vi "Galvo Module_sync.vi"(5 "sample mode":i32(ring)=10178 items=["Finite Samples"=10178, "Continuous Samples"=10123, "Hardware Timed Single Point"=12522], 7 "Action":T23=enum."Init: Calc scan pattern", 8 "error in (no error)":errorcluster, 10 "System Parameters":T1={"Optical Parameters"={"Obj. Focal Length [mm]"=45.0, "Scan Lens EFL[mm]"=60.0, "Tube Lens EFL[mm]"=180.0, "Galvo V Range (+/-)"=10.0, "Galvo Max Half Angle [Deg]"=19.0, "Max Galvo Range[%]"=0.0}, "Vibratome"={"Pre Cut Dwell [s]"=0.0, "Blade Frequency [RPM]"=0, "Slice Speed [mm/s]"=0.0, "Post Cut Dwell [s]"=0.0, "Ramp Time [s]"=0.0, "Start X [mm]"=0.0, "Start Y [mm]"=0.0, "Slice Length [mm]"=0.0, "Slice Axis"=enum."Y Axis", "Controller VISA Ref"="COM4"}, "Table Stages"={"X Stage"={"Position"=0.0, "Is.Enabled?"=FALSE, "Is.Connected?"=FALSE, "Device SN"="45876539", "AccelerationMaximum"=0.0, "VelocityMaximum"=0.0, "Acceleration"=0.0, "Velocity"=0.0, "waitTimeout (ms)"=0, "Model"=enum."None", "Is.Homed?"=FALSE, "MOVE"=FALSE}, "Y Stage"={"Position"=0.0, "Is.Enabled?"=FALSE, "Is.Connected?"=FALSE, "Device SN"="45876539", "AccelerationMaximum"=0.0, "VelocityMaximum"=0.0, "Acceleration"=0.0, "Velocity"=0.0, "waitTimeout (ms)"=0, "Model"=enum."None", "Is.Homed?"=FALSE, "MOVE"=FALSE}, "Z Stage"={"Position"=0.0, "Is.Enabled?"=FALSE, "Is.Connected?"=FALSE, "Device SN"="45876539", "AccelerationMaximum"=0.0, "VelocityMaximum"=0.0, "Acceleration"=0.0, "Velocity"=0.0, "waitTimeout (ms)"=0, "Model"=enum."None", "Is.Homed?"=FALSE, "MOVE"=FALSE}, "Attenuator"={"Position"=0.0, "Is.Enabled?"=FALSE, "Is.Connected?"=FALSE, "Device SN"="45876539", "AccelerationMaximum"=0.0, "VelocityMaximum"=0.0, "Acceleration"=0.0, "Velocity"=0.0, "waitTimeout (ms)"=0, "Model"=enum."None", "Is.Homed?"=FALSE, "MOVE"=FALSE}}, "Imaging Parameter"={"Raster Scan Direction"=enum."Uni Directional", "Pixel Dwell Time [Clock Cycles]"=1, "Flyback Time [Clock Cycles]"=10, "XY Center [um]"={"X"=1.0, "Y"=1.0}, "Pixel Step Size [um] X"=50.0, "XY Image Size"=enum."256 x 256", "Custom"=TRUE, "Custom Size"={"X"=10, "Y"=10}, "Line Averages"=1, "Pixel Step Size [um] Y"=0.0}, "Galvo HW Parameters"={"Analog Out Channel"="GalvoCtrl/ao0,GalvoCtrl/ao1", "Min Voltage"=-10.0, "Max Voltage"=10.0, "Pixel Clock Source"="/GalvoCtrl/PFI0", "Sample Rate"=1000.0, "Line Clock Out Ch"="GalvoCtrl/port0/line0", "2P ready check"="GalvoCtrl/port0/line0"}, "Alazar parameters"={"Trigger Settings"={"General Trigger Settings"={"Trigger Operation"=0, "Coupling ID"=2, "Range ID"=2, "Delay"=0, "Timeout Ticks"=0, "Mode"=1, "Parameter"=1}, "Trigger Engine 1"={"Trigger Engine"=0, "Source"=2, "Slope"=1, "Level"=140}, "Trigger Engine 2"={"Trigger Engine"=1000, "Source"=4294967295, "Slope"=1, "Level"=2048}}, "Device ID"={"System ID"=1, "Board ID"=1}, "Ch A Input Control"={"Channel"=1, "Coupling"=2, "Range"=10, "Impedance"=2}, "Ch B Input Control"={"Channel"=2, "Coupling"=2, "Range"=10, "Impedance"=2}, "Acq Settings"={"Record Length"=1440, "Offset"=0, "Records Per Buffer"=2048, "Records Count (Records/Acq)"=2147483647, "Window Type"=1, "Footer"=0, "Samples per record"=2048, "Output Format"=257}, "Capture Clock"={"Sample Rate"=100, "Decimation"=0, "Source"=2, "Edge"=0}}, "Mosaic Paramter"={"X Axis"={"Start [mm]"=0.0, "Steps [pts]"=0.0, "End [mm]"=0.0}, "Y Axis"={"Start [mm]"=0.0, "Steps [pts]"=0.0, "End [mm]"=0.0}, "Scan Pattern"=enum."Uni-directional", "Overlap Options"={"Overlap Type"=enum."No Overlap", "Percent Overlap"=0, "Justify"=enum."Start"}}, "Manual Controls"={"Data Path"=path "", "Save parameters"={"start pixel"=45, "#pixels to save"=100}, "Acquisition mode"=enum."Alazar FFT", "PSOCT Channel"=1, "Save data?"=FALSE, "AIP rotation angle"=0.0, "Outgoing Mail Server (SMTP)"="smtp.gmail.com", "Email"="", "Password"="", "Carrier 1"=enum."Sprint", "phone number 1"="", "Subject"="", "Message"="", "Carrier 2"=enum."Sprint", "phone number 2"="", "Outputs for GPU FFT"=enum."Amp + Phase diff", "First Slice #"=1}, "Z stage setting"={"first cut height(mm)"=45.85, "cut thickness[um]"=[], "#cycles"=111, "PSOCT thickness(um)"=[], "First image height(mm)"=2.1, "Pause?"=[], "Z0"=0.0, "fixed Z0?"=FALSE, "Cut_aft_2P?(leave empty if no 2P)"=[], "2P thickness(um) (leave empty if not used)"=[], "2P_cover_all_depth? (leave empty if no 2P)"=[]}, "Attenuator"={"Power after Objective (recalibrate every 6 month)"=[]}, "Pause?"=FALSE} {"Manual Controls"."PSOCT Channel" items=["A"=1, "B"=2, "A + B"=3, "C"=4, "A + C"=5, "A + B"=6, "D"=8, "A + D"=9, "B + D"=10, "C + D"=12, "A + B + C + D"=15]; "Alazar parameters"."Capture Clock"."Edge" items=["Rising", "Falling"]; "Alazar parameters"."Capture Clock"."Source" items=["Internal"=1, "Fast External"=2, "Medium External"=3, "Slow External"=4, "External AC"=5, "External DC"=6, "External 10MHz"=7]; "Alazar parameters"."Acq Settings"."Output Format" items=["Float Log"=11, "Float Amp"=10, "U16_LOG"=1, "U16_AMP2"=257, "Real"=3, "Imag"=4]; "Alazar parameters"."Acq Settings"."Footer" items=["FOOTER_NONE", "FOOTER_NPT"]; "Alazar parameters"."Acq Settings"."Window Type" items=["DSP_WINDOW_NONE", "DSP_WINDOW_HANNING", "DSP_WINDOW_HAMMING", "DSP_WINDOW_BLACKMAN", "DSP_WINDOW_BLACKMAN_HARRIS", "DSP_WINDOW_BARTLETT"]; "Alazar parameters"."Ch B Input Control"."Channel" items=["A"=1, "B"=2, "C"=4, "D"=8]; "Alazar parameters"."Ch B Input Control"."Coupling" items=["AC"=1, "DC"=2]; "Alazar parameters"."Ch B Input Control"."Range" items=["20 mV"=1, "40 mV"=2, "50 mV"=3, "80 mV"=4, "100 mV"=5, "200 mV"=6, "400 mV"=7, "500 mV"=8, "800 mV"=9, "1 V"=10, "1.25 V"=33, "2 V"=11, "4 V"=12, "5 V"=13, "8 V"=14, "10 V"=15, "20 V"=16]; "Alazar parameters"."Ch B Input Control"."Impedance" items=["1 MOhm"=1, "50 Ohm"=2, ""=0]; "Alazar parameters"."Ch A Input Control"."Channel" items=["A"=1, "B"=2, "C"=4, "D"=8]; "Alazar parameters"."Ch A Input Control"."Coupling" items=["AC"=1, "DC"=2]; "Alazar parameters"."Ch A Input Control"."Range" items=["20 mV"=1, "40 mV"=2, "50 mV"=3, "80 mV"=4, "100 mV"=5, "200 mV"=6, "400 mV"=7, "500 mV"=8, "800 mV"=9, "1 V"=10, "1.25 V"=33, "2 V"=11, "4 V"=12, "5 V"=13, "8 V"=14, "10 V"=15, "20 V"=16]; "Alazar parameters"."Ch A Input Control"."Impedance" items=["1 MOhm"=1, "50 Ohm"=2, ""=0]; "Alazar parameters"."Trigger Settings"."General Trigger Settings"."Trigger Operation" items=["J", "K", "J OR K", "J AND K", "J XOR K", "J AND NOT K", "NOT J AND K"]; "Alazar parameters"."Trigger Settings"."General Trigger Settings"."Coupling ID" items=["AC"=1, "DC"=2]; "Alazar parameters"."Trigger Settings"."General Trigger Settings"."Range ID" items=["5 V", "1 V", "TTL"]; "Alazar parameters"."Trigger Settings"."Trigger Engine 1"."Trigger Engine" items=["J", "K"]; "Alazar parameters"."Trigger Settings"."Trigger Engine 1"."Source" items=["A", "B", "External", "Disable", "C", "D"]; "Alazar parameters"."Trigger Settings"."Trigger Engine 1"."Slope" items=["Positive"=1, "Negative"=2]; "Alazar parameters"."Trigger Settings"."Trigger Engine 2"."Trigger Engine" items=["J", "K"]; "Alazar parameters"."Trigger Settings"."Trigger Engine 2"."Source" items=["A", "B", "External", "Disable", "C", "D"]; "Alazar parameters"."Trigger Settings"."Trigger Engine 2"."Slope" items=["Positive"=1, "Negative"=2]; "Imaging Parameter"."Pixel Step Size [um] Y" min=0.0 max=100.0 step=0.01; "Imaging Parameter"."Line Averages" min=1 max=30 step=1; "Imaging Parameter"."Flyback Time [Clock Cycles]" max=10 step=1; "Imaging Parameter"."Pixel Step Size [um] X" min=0.0 max=100.0 step=0.01; "Imaging Parameter"."Custom Size"."Y" min=1 max=30 step=1; "Imaging Parameter"."Custom Size"."X" min=1 max=30 step=1; "Imaging Parameter"."XY Center [um]"."Y" min=1.0 max=30.0 step=1.0; "Imaging Parameter"."XY Center [um]"."X" min=1.0 max=30.0 step=1.0; "Imaging Parameter"."Pixel Dwell Time [Clock Cycles]" max=10 step=1}) -> (0 "error out":errorcluster, 1 "task done?":bool)   [LabVIEW 2018]
uses:
  type defines/Galvo controls.ctl
  Controls/System Parameters.ctl
  Controls/Optical Parameters.ctl
  Controls/Vibratome Parameters.ctl
  Controls/Translation Stage Parameters.ctl
  Hardware Mfg/Thorlabs Translation Stages/Controls/Translation Stage Cluster.ctl
  Controls/Translation Stage Types.ctl
  Controls/Imaging Parameters.ctl
  Controls/Scan Direction.ctl
  type defines/Alazar parameters.ctl
  Hardware Mfg/AlazarTech SDK/Controls/General Trigger Settings.ctl
  Hardware Mfg/AlazarTech SDK/Controls/Trigger Engine Controls.ctl
  Hardware Mfg/AlazarTech SDK/Controls/Alazar Device ID.ctl
  Hardware Mfg/AlazarTech SDK/Controls/Channel Input Controls.ctl
  Hardware Mfg/AlazarTech SDK/Controls/Alazar Acquisition Settings.ctl
  Hardware Mfg/AlazarTech SDK/Controls/Clock Controls.ctl
  type defines/Mosaic Parameter.ctl
  type defines/Manual Controls.ctl
  type defines/FFT parameters.ctl
  type defines/FFT mode.ctl
  type defines/GPU FFT outputs.ctl
  type defines/Vibratome Param.ctl
  type defines/attenuator.ctl
  <vilib>/DAQmx/write.llb/DAQmx Write (Digital 1D U32 1Chan NSamp).vi
  <vilib>/DAQmx/write.llb/DAQmx Write (Analog 2D DBL NChan NSamp).vi
  <vilib>/DAQmx/create/channels.llb/DAQmx Create Channel (CO-Pulse Generation-Time).vi
  <vilib>/DAQmx/create/channels.llb/DAQmx Create Channel (AO-Voltage-Basic).vi
  <vilib>/DAQmx/configure/timing.llb/DAQmx Timing (Sample Clock).vi
  <vilib>/DAQmx/create/channels.llb/DAQmx Create Channel (DO-Digital Output).vi
  <vilib>/DAQmx/configure/trigger.llb/DAQmx Start Trigger (Digital Edge).vi
  <vilib>/DAQmx/miscellaneous.llb/DAQmx Fill In Error Info.vi
  <resource>/objmgr/daqmx.rc
panel:
  # "X"
  # "X"
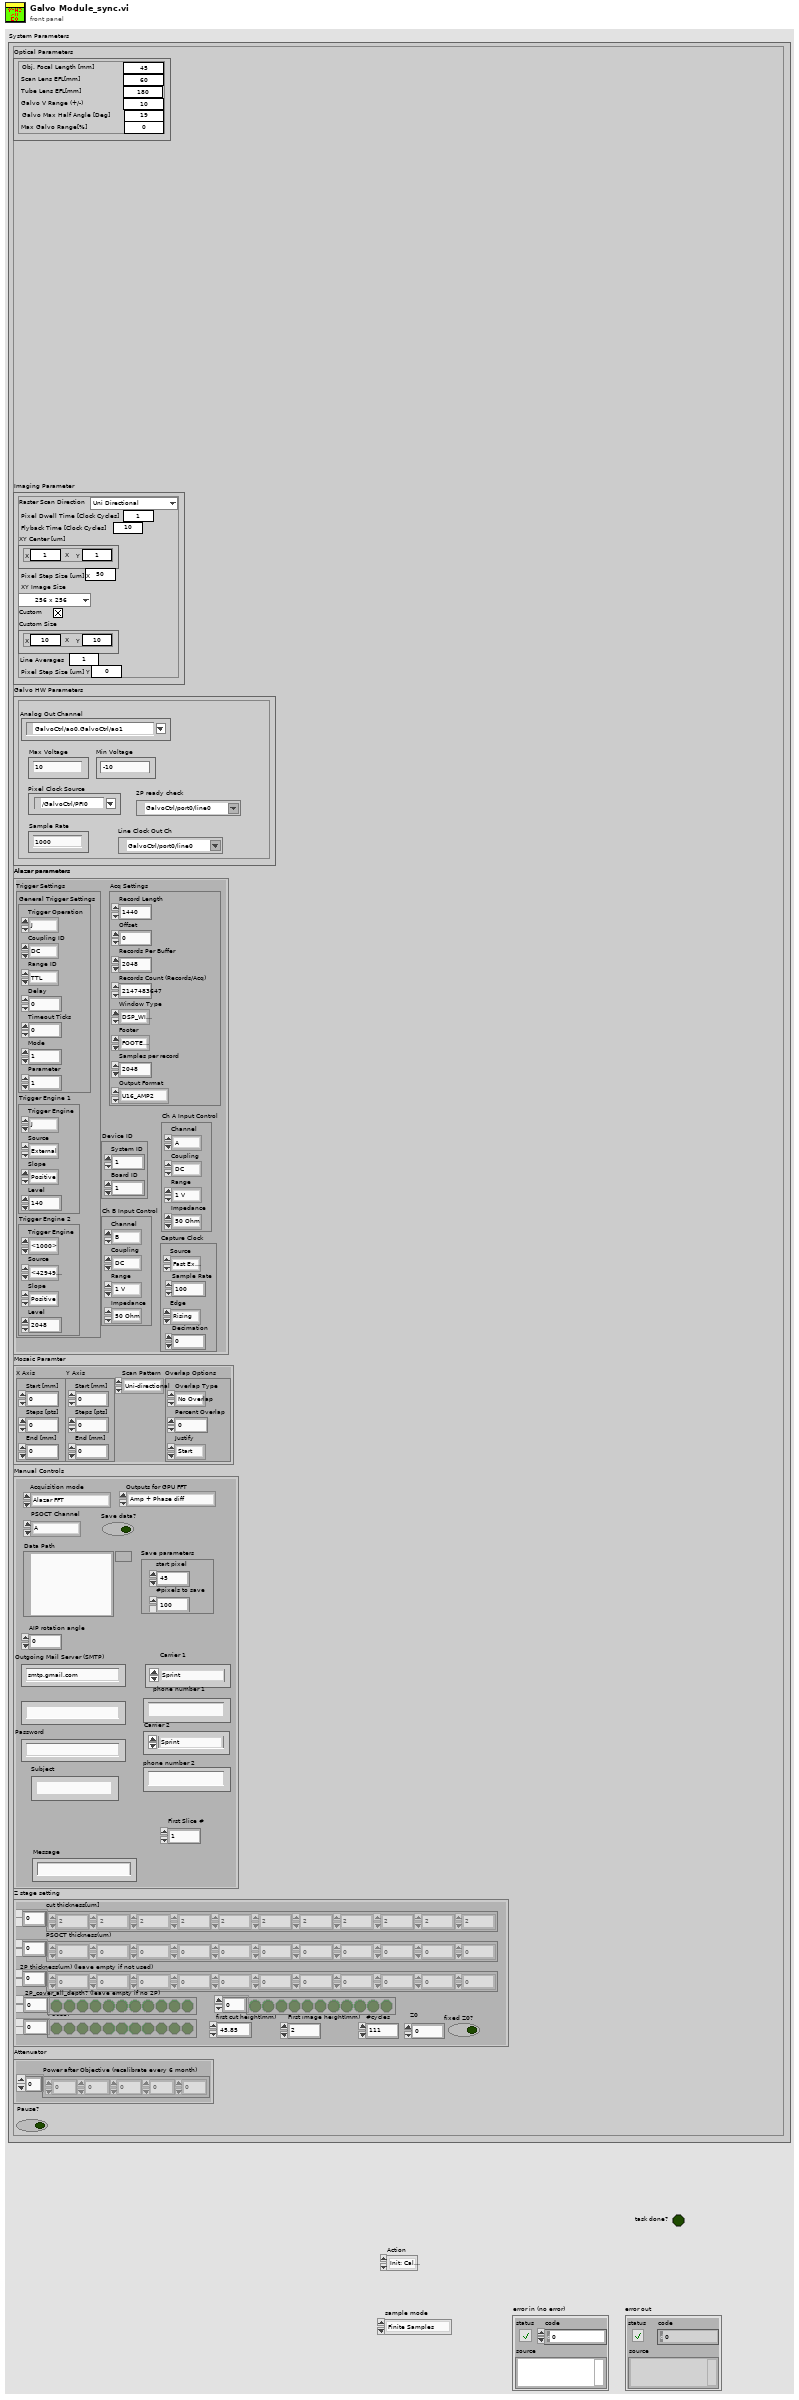
[diagram p1: front panel]
types:
  T1 = typedef "System Parameters.ctl" = cluster{"Optical Parameters":T2, "Vibratome":T3, "Table Stages":T4, "Imaging Parameter":T7, "Galvo HW Parameters":cluster{"Analog Out Channel":tag, "Min Voltage":dbl, "Max Voltage":dbl, "Pixel Clock Source":tag, "Sample Rate":dbl, "Line Clock Out Ch":tag, "2P ready check":tag}, "Alazar parameters":T9, "Mosaic Paramter":T16, "Manual Controls":T17, "Z stage setting":T21, "Attenuator":T22, "Pause?":bool}
  T2 = typedef "Optical Parameters.ctl" = cluster{"Obj. Focal Length [mm]":dbl, "Scan Lens EFL[mm]":dbl, "Tube Lens EFL[mm]":dbl, "Galvo V Range (+/-)":dbl, "Galvo Max Half Angle [Deg]":dbl, "Max Galvo Range[%]":dbl}
  T3 = typedef "Vibratome Parameters.ctl" = cluster{"Pre Cut Dwell [s]":dbl, "Blade Frequency [RPM]":u16, "Slice Speed [mm/s]":dbl, "Post Cut Dwell [s]":dbl, "Ramp Time [s]":dbl, "Start X [mm]":dbl, "Start Y [mm]":dbl, "Slice Length [mm]":dbl, "Slice Axis":enum16{"X Axis", "Y Axis", "Z Axis"}, "Controller VISA Ref":refnum<visa-resource-name>}
  T4 = typedef "Translation Stage Parameters.ctl" = cluster{"X Stage":T5, "Y Stage":T5, "Z Stage":T5, "Attenuator":T5}
  T5 = typedef "Translation Stage Cluster.ctl" = cluster{"Position":dbl, "Is.Enabled?":bool, "Is.Connected?":bool, "Device SN":string, "AccelerationMaximum":dbl, "VelocityMaximum":dbl, "Acceleration":dbl, "Velocity":dbl, "waitTimeout (ms)":i32, "Model":T6, "Is.Homed?":bool, "MOVE":bool}
  T6 = typedef "Translation Stage Types.ctl" = enum16{"None", "Thorlabs LTS", "Thorlabs MLJ"}
  T7 = typedef "Imaging Parameters.ctl" = cluster{"Raster Scan Direction":T8, "Pixel Dwell Time [Clock Cycles]":u16, "Flyback Time [Clock Cycles]":u16, "XY Center [um]":cluster{"X":dbl, "Y":dbl}, "Pixel Step Size [um] X":dbl, "XY Image Size":enum16{"32 x 32", "64 x 64", "128 x 128", "256 x 256", "512 x 512", "1024 x 1024", "2048 x 2048"}, "Custom":bool, "Custom Size":cluster{"X":u16, "Y":u16}, "Line Averages":u16, "Pixel Step Size [um] Y":dbl}
  T8 = typedef "Scan Direction.ctl" = enum16{"Uni Directional", "Bi Directional", "None"}
  T9 = typedef "Alazar parameters.ctl" = cluster{"Trigger Settings":cluster{"General Trigger Settings":T10, "Trigger Engine 1":T11, "Trigger Engine 2":T11}, "Device ID":T12, "Ch A Input Control":T13, "Ch B Input Control":T13, "Acq Settings":T14, "Capture Clock":T15}
  T10 = typedef "General Trigger Settings.ctl" = cluster{"Trigger Operation":u32, "Coupling ID":u32, "Range ID":u32, "Delay":u32, "Timeout Ticks":u32, "Mode":u32, "Parameter":u32}
  T11 = typedef "Trigger Engine Controls.ctl" = cluster{"Trigger Engine":u32, "Source":u32, "Slope":u32, "Level":u32}
  T12 = typedef "Alazar Device ID.ctl" = cluster{"System ID":u32, "Board ID":u32}
  T13 = typedef "Channel Input Controls.ctl" = cluster{"Channel":u8, "Coupling":u32, "Range":u32, "Impedance":u32}
  T14 = typedef "Alazar Acquisition Settings.ctl" = cluster{"Record Length":u32, "Offset":u32, "Records Per Buffer":u32, "Records Count (Records/Acq)":u32, "Window Type":u32, "Footer":u32, "Samples per record":u32, "Output Format":u32}
  T15 = typedef "Clock Controls.ctl" = cluster{"Sample Rate":u32, "Decimation":u32, "Source":u32, "Edge":u32}
  T16 = typedef "Mosaic Parameter.ctl" = cluster{"X Axis":cluster{"Start [mm]":dbl, "Steps [pts]":dbl, "End [mm]":dbl}, "Y Axis":cluster{"Start [mm]":dbl, "Steps [pts]":dbl, "End [mm]":dbl}, "Scan Pattern":enum16{"Uni-directional", "Bi-Directional", "Spiral Out", "Spiral In"}, "Overlap Options":cluster{"Overlap Type":enum16{"No Overlap", "X Only", "Y Only", "X and Y"}, "Percent Overlap":u8, "Justify":enum16{"Start", "Center", "End"}}}
  T17 = typedef "Manual Controls.ctl" = cluster{"Data Path":path, "Save parameters":T18, "Acquisition mode":T19, "PSOCT Channel":u32, "Save data?":bool, "AIP rotation angle":dbl, "Outgoing Mail Server (SMTP)":string, "Email":string, "Password":string, "Carrier 1":enum16{"T-Mobile", "AT&T", "Verizon", "Sprint"}, "phone number 1":string, "Subject":string, "Message":string, "Carrier 2":enum16{"T-Mobile", "AT&T", "Verizon", "Sprint"}, "phone number 2":string, "Outputs for GPU FFT":T20, "First Slice #":i32}
  T18 = typedef "FFT parameters.ctl" = cluster{"start pixel":i32, "#pixels to save":i32}
  T19 = typedef "FFT mode.ctl" = enum16{"ThorOCT B line", "ThorOCT Spectral", "ThorOCT FFT", "Alazar B line", "Alazar FFT", "GPU FFT", "Alazar Spectral", "Simulation", "auto adjust focus", "Save all"}
  T20 = typedef "GPU FFT outputs.ctl" = enum16{"Amp + Phase diff", "Amp + Phase", "Amp only"}
  T21 = typedef "Vibratome Param.ctl" = cluster{"first cut height(mm)":dbl, "cut thickness[um]":u32[], "#cycles":u16, "PSOCT thickness(um)":u32[], "First image height(mm)":dbl, "Pause?":bool[], "Z0":dbl, "fixed Z0?":bool, "Cut_aft_2P?(leave empty if no 2P)":bool[], "2P thickness(um) (leave empty if not used)":u32[], "2P_cover_all_depth? (leave empty if no 2P)":bool[]}
  T22 = typedef "attenuator.ctl" = cluster{"Power after Objective (recalibrate every 6 month)":dbl[]}
  T23 = typedef "Galvo controls.ctl" = enum16{"Configure channels", "Write Scan Pattern", "Start Galvo Task", "Is Task Done?", "Stop Galvo", "Uninit", "Init: Calc scan pattern", "Start DO only", "Uninit DO only", "Write DO only", "Configure DO only", "Zero arrays", "write zero array DO"}
  T24 = cluster{"Analog Out Channel":tag, "Min Voltage":dbl, "Max Voltage":dbl, "Pixel Clock Source":tag, "Sample Rate":dbl, "Line Clock Out Ch":tag, "2P ready check":tag}
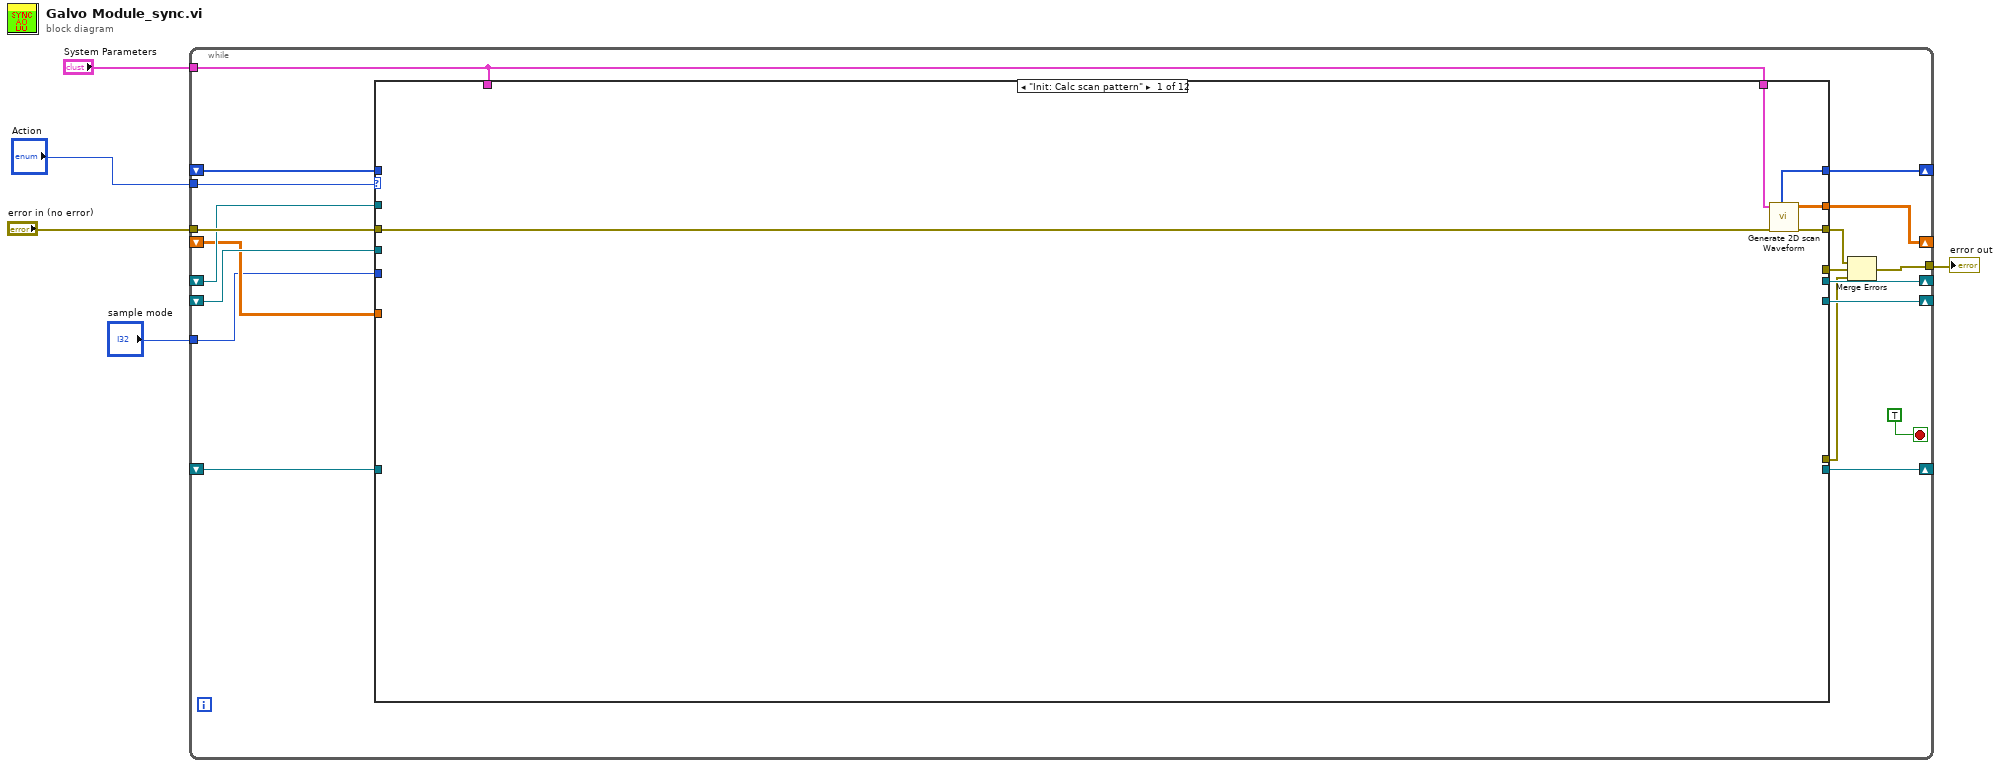
[diagram p0: block diagram]
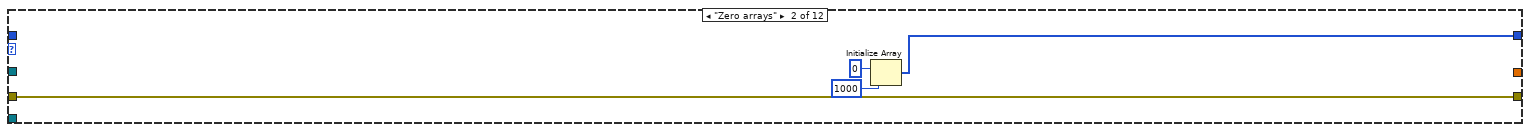
[diagram p2: hidden frame]
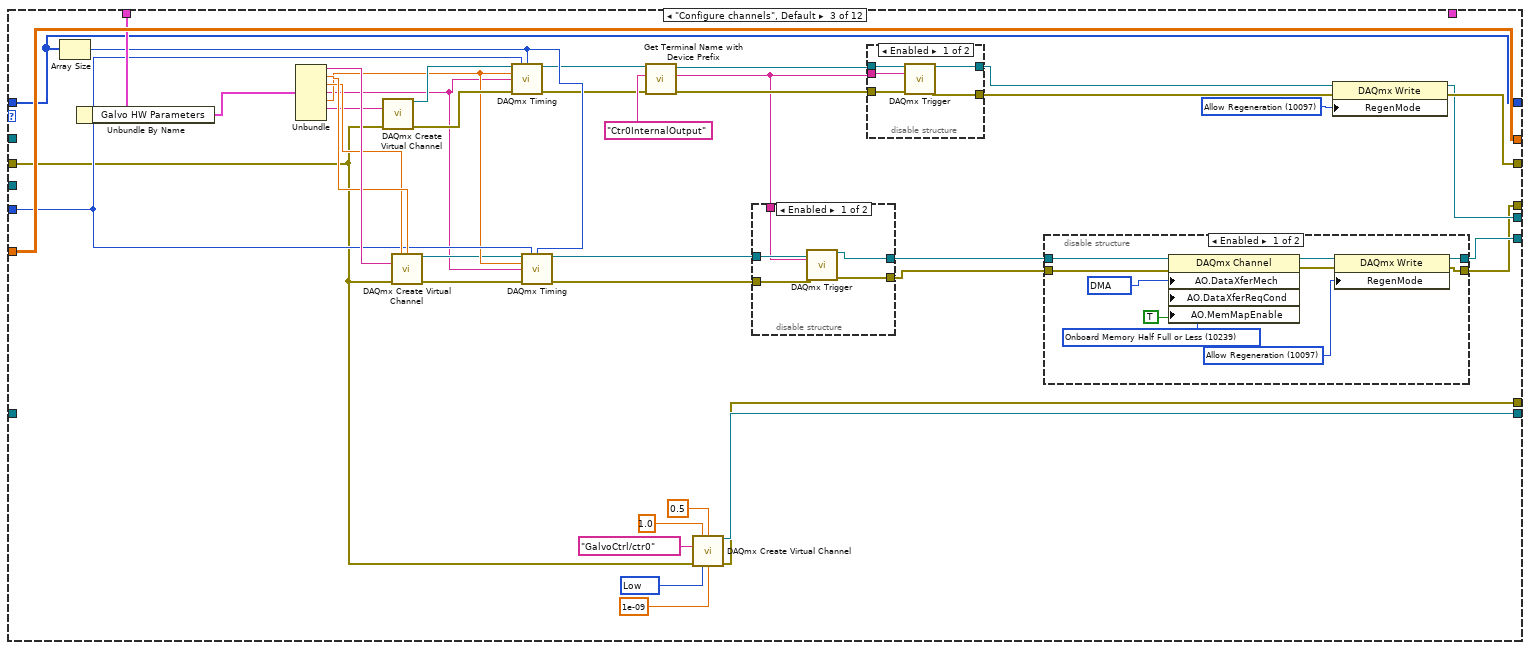
[diagram p3: hidden frame]
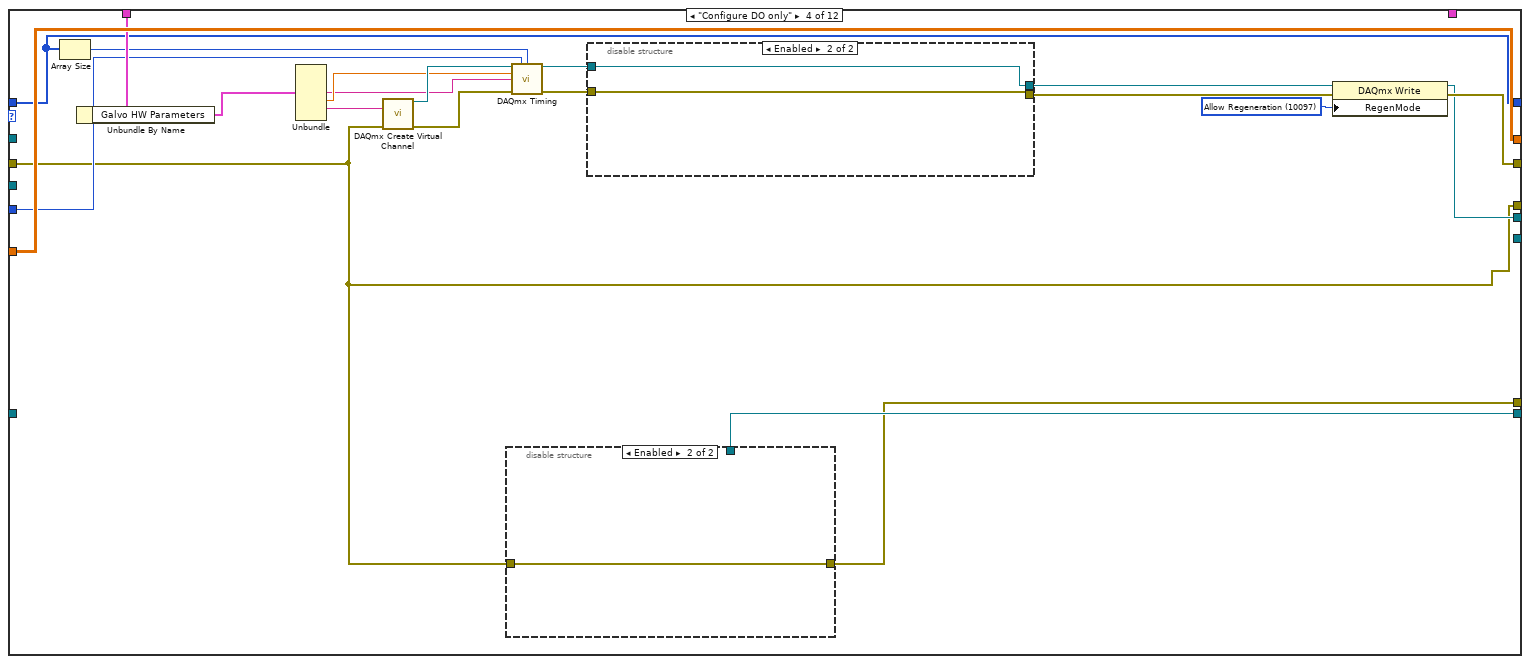
[diagram p7: hidden frame]
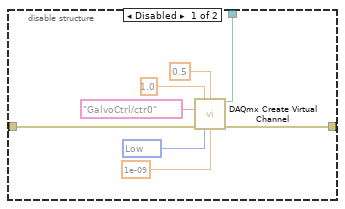
[diagram p8: hidden frame]
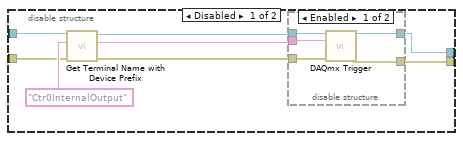
[diagram p9: hidden frame]
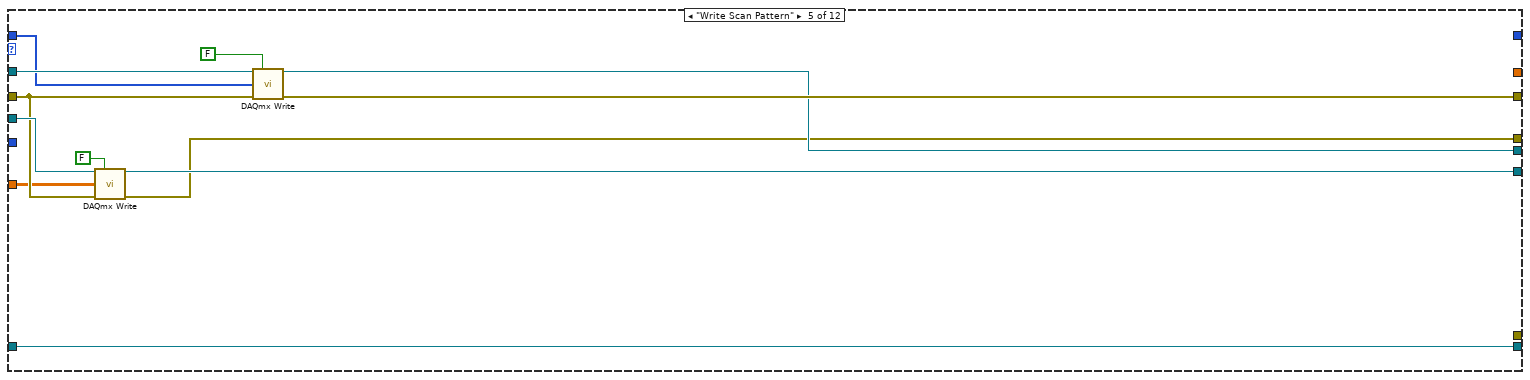
[diagram p11: hidden frame]
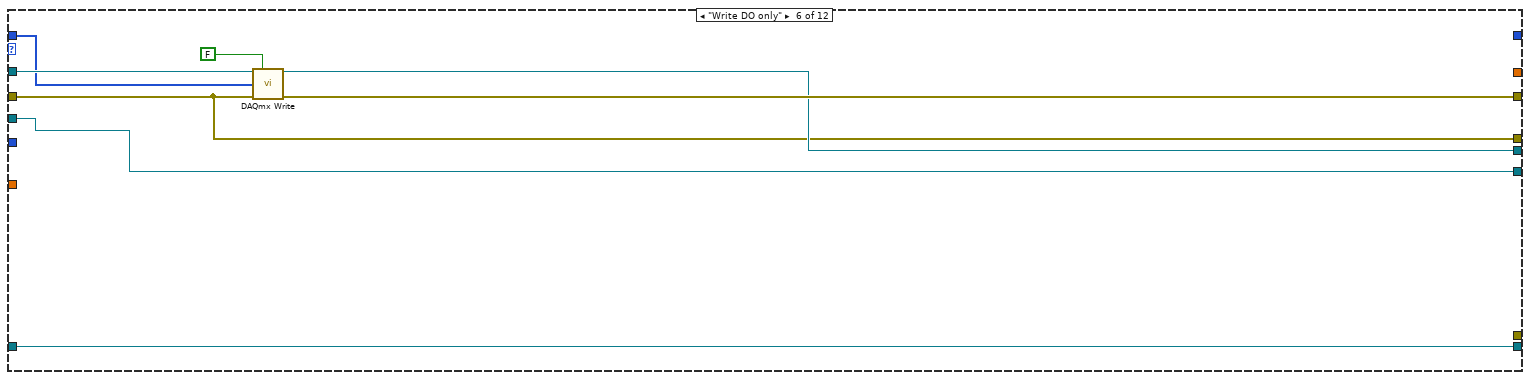
[diagram p12: hidden frame]
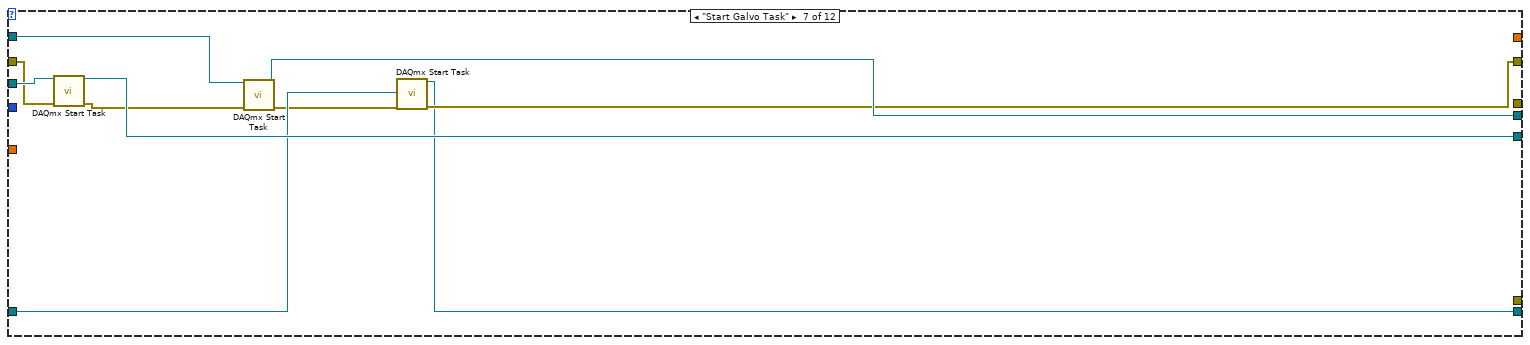
[diagram p13: hidden frame]
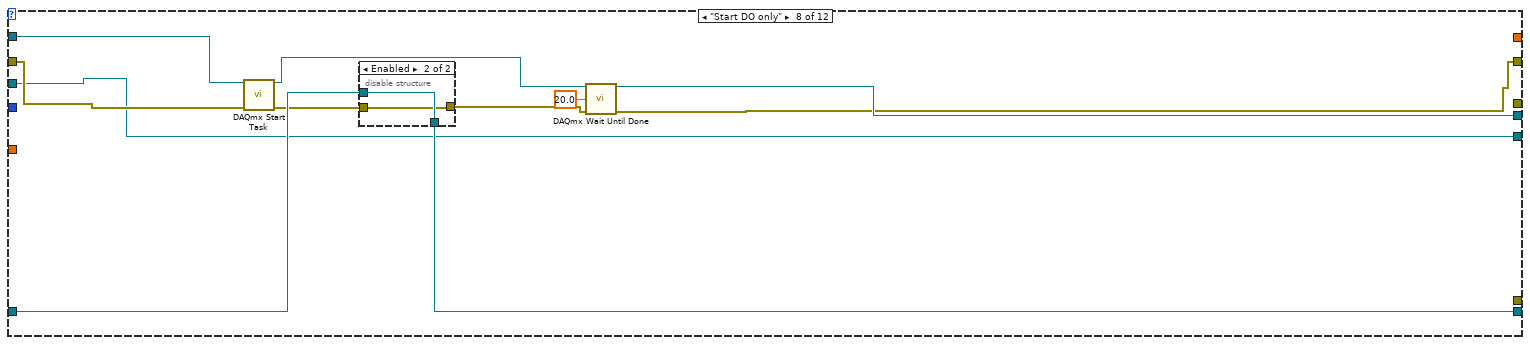
[diagram p14: hidden frame]
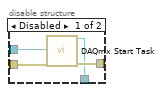
[diagram p15: hidden frame]
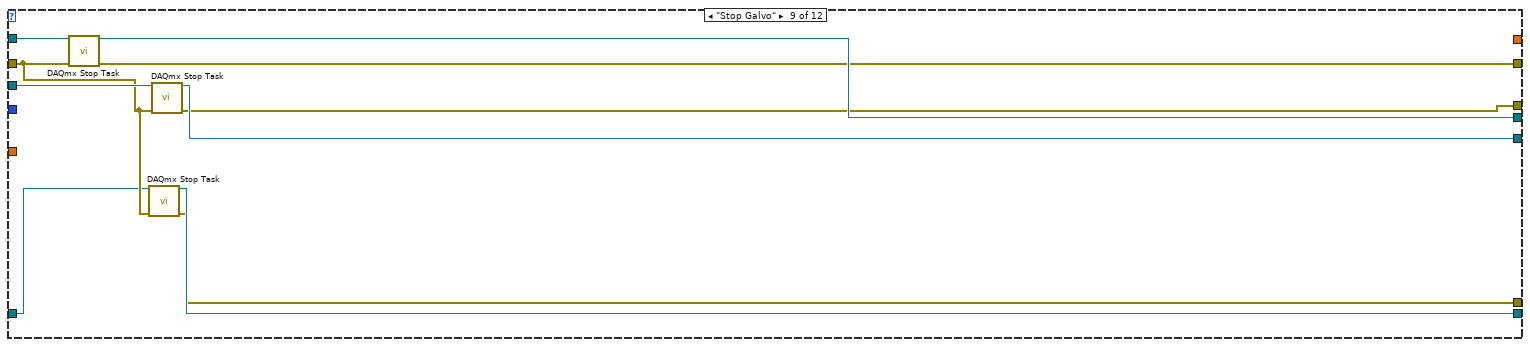
[diagram p16: hidden frame]
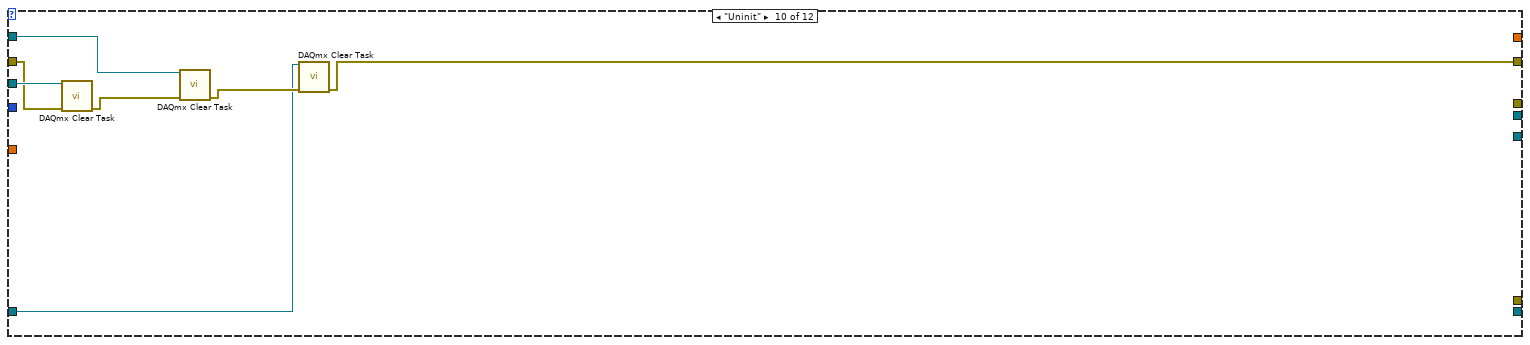
[diagram p17: hidden frame]
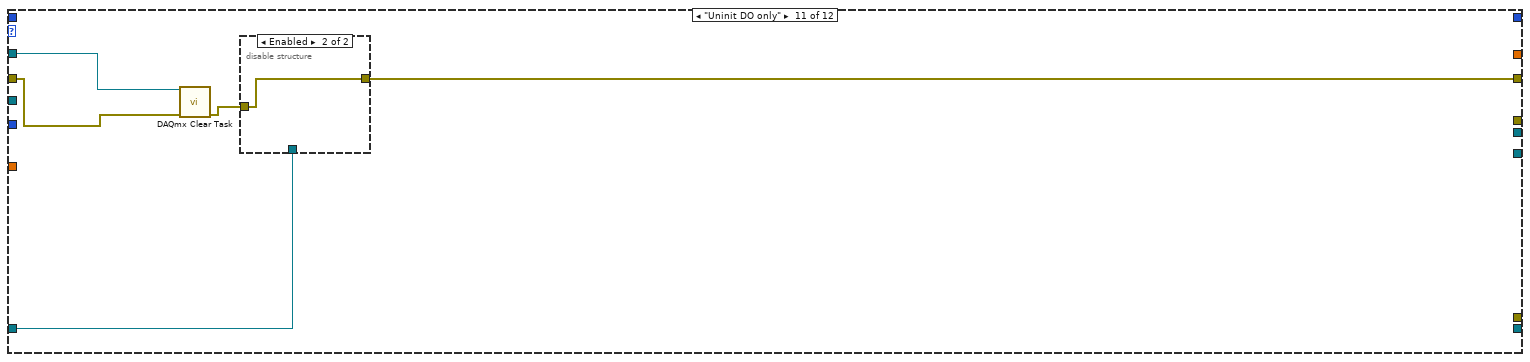
[diagram p18: hidden frame]
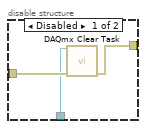
[diagram p19: hidden frame]
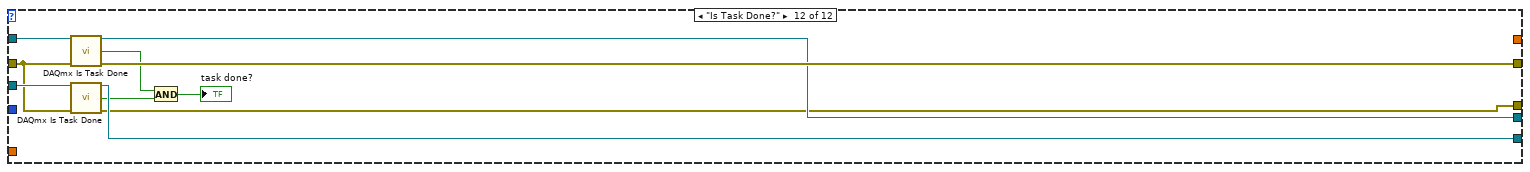
[diagram p20: hidden frame]
diagram:
  n1 = while {
    tunnel: "Action" -> [w24]
    shift-right: [w23] -> _
    shift-left: _ -> [w22]
    tunnel: [w19] -> w4
    tunnel: "error in (no error)" -> [w21]
    shift-right: [w17] -> _
    shift-left: _ -> [w16]
    shift-right: [w15] -> _
    shift-left: _ -> [w14]
    tunnel: "sample mode" -> [w13]
    tunnel: "System Parameters" -> [w11]
    shift-right: [w10] -> _
    shift-left: _ -> [w9]
    shift-right: [w8] -> _
    shift-left: _ -> [w7]
    stop <- TRUE stop-if-true
    n2 = case shown="\"Init: Calc scan pattern\"" w24 {
      tunnel: [_ _ w71 _ w153 w161 w176 w183 w203 _ _ w229] -> w23
      tunnel: w22 -> [_ _ _ _ w159 w161 w177 w183 w204 w211 _ w230]
      tunnel: w21 -> [w27 w33 w50 w101 w158 w160 w173 w184 w198 w209 w212 w221]
      tunnel: [w28 w33 w67 w118 w157 w167 w169 w179 w200 w206 w214 w226] -> w18
      tunnel: [_ _ w66 w117 w155 w165 w174 w181 w201 _ _ w223] -> w17
      tunnel: w16 -> [_ _ _ _ w154 w164 w175 w188 w202 w210 w216 w227]
      tunnel: [w29 _ w65 w116 _ _ _ _ _ _ _ _] -> w15
      tunnel: w14 -> [_ _ w65 w116 w152 _ _ _ _ _ _ _]
      tunnel: w13 -> [_ _ w61 w113 _ _ _ _ _ _ _ _]
      tunnel: [_ _ w64 w101 w151 w160 _ _ w199 _ _ w222] -> w12
      tunnel: w11 -> [w26 _ _ _ _ _ _ _ _ _ _ _]
      tunnel: w11 -> [_ _ w63 w115 _ _ _ _ _ _ _ _]
      tunnel: [w25 w30 w58 w110 _ _ _ _ _ _ _ _] -> w10
      tunnel: w9 -> [_ _ w58 w110 w150 w163 _ _ _ _ _ _]
      tunnel: [_ _ w42 w107 w148 w162 w168 w185 w196 _ _ _] -> w8
      tunnel: w7 -> [_ _ _ _ w148 w162 w171 w187 w197 w205 w213 _]
      tunnel: [_ _ w41 w106 _ _ _ _ w195 _ _ _] -> w6
      frame "Init: Calc scan pattern" {
        n3 = call "Generate 2D scan Waveform.vi"("error in (no error)"=w27, "System Parameters [In]"=w26) -> ("error out"=w28:errorcluster, "XY"=w29:dbl[][], "DO"=w25:u32[])  [unwired: 3 in, 4 out]
      }
      frame "Zero arrays" {
        n4 = Initialize Array(u32 0 ("element"), 1000 ("dimension size")) -> (w30:u32[])
      }
      frame "Configure channels", Default {
        w34 = 10097 items=["Allow Regeneration"=10097, "Do Not Allow Regeneration"=10158] ("RegenMode")
        w55 = 10214 items=["High"=10192, "Low"=10214] ("Idle State")
        n5 = Array Size(array=w58) -> (size(s)=w60:i32)
        n6 = Unbundle By Name(w63) -> ("Galvo HW Parameters"=w62:T24)
        n7 = Unbundle(w62) -> ("Analog Out Channel"=w74:tag, "Min Voltage"=w73:dbl, "Max Voltage"=w72:dbl, "Pixel Clock Source"=w40:tag, "Sample Rate"=w59:dbl, "Line Clock Out Ch"=w70:tag)  [unwired: 1 out]
        n8 = call-poly <vilib>:"DAQmx Create Virtual Channel.vi"("lines"=w70, "error in"=w50) -> ("task out"=w68:refnum<k21>, "error out"=w69:errorcluster)  [unwired: 12 in]
        n9 = call-poly <vilib>:"DAQmx Create Virtual Channel.vi"("maximum value"=w72, "minimum value"=w73, "physical channels"=w74, "error in"=w50) -> ("task out"=w57:refnum<k21>, "error out"=w56:errorcluster)  [unwired: 10 in]
        n10 = call-poly <vilib>:"DAQmx Timing.vi"("task/channels in"=w68, "sample mode"=w61, "samples per channel"=w60, "rate"=w59, "source"=w40, "error in"=w69) -> ("task out"=w47:refnum<k21>, "error out"=w48:errorcluster)  [unwired: 8 in]
        n11 = call-poly <vilib>:"DAQmx Timing.vi"("task/channels in"=w57, "sample mode"=w61, "samples per channel"=w60, "rate"=w59, "source"=w40, "error in"=w56) -> ("task out"=w44:refnum<k21>, "error out"=w46:errorcluster)  [unwired: 8 in]
        n12 = call "Get Terminal Name with Device Prefix.vi"("error in (no error)"=w48, "Local Terminal Name"="Ctr0InternalOutput" ("terminal"), "task/channels in"=w47) -> ("error out"=w39:errorcluster, "Terminal Name with Device Prefix"=w35:tag, "task out"=w38:refnum<k21>)  [unwired: 1 in, 5 out]
        n13 = call-poly <vilib>:"DAQmx Create Virtual Channel.vi"("high time"=1.0 ("High Time"), "low time"=0.5 ("Low Time"), "counter"=tag "GalvoCtrl/ctr0" ("Counter(s)"), "error in"=w50, "idle state"=w55, "initial delay"=1e-09 ("Initial Delay")) -> ("task out"=w42:refnum<k21>, "error out"=w41:errorcluster)  [unwired: 3 in, 5 out]
        n14 = disable-structure shown="Enabled" {
          disable-tunnel: w46 -> [w86 w87]
          disable-tunnel: [w85 w87] -> w45
          disable-tunnel: w44 -> [w84 w88]
          disable-tunnel: [w83 w88] -> w43
          disable-tunnel: w35 -> [w82 _]
          frame Enabled {
            n15 = call-poly <vilib>:"DAQmx Trigger.vi"("task/channels in"=w84, "source"=w82, "error in"=w86) -> ("task out"=w83:refnum<k21>, "error out"=w85:errorcluster)  [unwired: 2 in, 9 out]
          }
          frame Disabled {
          }
        }
        n16 = disable-structure shown="Enabled" {
          disable-tunnel: w39 -> [w79 w81]
          disable-tunnel: w38 -> [w78 w80]
          disable-tunnel: [w77 w80] -> w37
          disable-tunnel: [w76 w81] -> w36
          disable-tunnel: w35 -> [w75 _]
          frame Enabled {
            n17 = call-poly <vilib>:"DAQmx Trigger.vi"("task/channels in"=w78, "source"=w75, "error in"=w79) -> ("task out"=w77:refnum<k21>, "error out"=w76:errorcluster)  [unwired: 2 in, 9 out]
          }
          frame Disabled {
          }
        }
        n18 = disable-structure shown="Enabled" {
          disable-tunnel: w45 -> [w98 w99]
          disable-tunnel: w43 -> [w96 w100]
          disable-tunnel: [w92 w99] -> w64
          disable-tunnel: [w89 w100] -> w71
          frame Enabled {
            w90 = 10097 items=["Allow Regeneration"=10097, "Do Not Allow Regeneration"=10158] ("RegenMode")
            w94 = 10239 items=["Onboard Memory Empty"=10235, "Onboard Memory Half Full or Less"=10239, "Onboard Memory Less than Full"=10242] ("AO.DataXferReqCond")
            w95 = 10054 items=["DMA"=10054, "Interrupts"=10204, "Programmed I/O"=10264, "USB Bulk"=12590] ("AO.DataXferMech")
            n19 = property class="DAQmx Channel"(reference=w96, error in=w98, "AO.DataXferMech"=w95, "AO.DataXferReqCond"=w94, "AO.MemMapEnable"=TRUE) -> (reference out=w91:refnum<k21>, error out=w97:errorcluster)
            n20 = property class="DAQmx Write"(reference=w91, error in=w97, "RegenMode"=w90) -> (reference out=w89:refnum<k21>, error out=w92:errorcluster)
          }
          frame Disabled {
          }
        }
        n21 = property class="DAQmx Write"(reference=w37, error in=w36, "RegenMode"=w34) -> (reference out=w66:refnum<k21>, error out=w67:errorcluster)
      }
      frame "Configure DO only" {
        w102 = 10097 items=["Allow Regeneration"=10097, "Do Not Allow Regeneration"=10158] ("RegenMode")
        n22 = Array Size(array=w110) -> (size(s)=w112:i32)
        n23 = Unbundle By Name(w115) -> ("Galvo HW Parameters"=w114:T24)
        n24 = Unbundle(w114) -> ("Pixel Clock Source"=w105:tag, "Sample Rate"=w111:dbl, "Line Clock Out Ch"=w121:tag)  [unwired: 4 out]
        n25 = call-poly <vilib>:"DAQmx Create Virtual Channel.vi"("lines"=w121, "error in"=w101) -> ("task out"=w119:refnum<k21>, "error out"=w120:errorcluster)  [unwired: 12 in]
        n26 = disable-structure shown="Enabled" {
          disable-tunnel: [w124 _] -> w107
          disable-tunnel: [w123 w130] -> w106
          disable-tunnel: w101 -> [w122 w130]
          frame Disabled {
            w129 = 10214 items=["High"=10192, "Low"=10214] ("Idle State")
            n27 = call-poly <vilib>:"DAQmx Create Virtual Channel.vi"("high time"=1.0 ("High Time"), "low time"=0.5 ("Low Time"), "counter"=tag "GalvoCtrl/ctr0" ("Counter(s)"), "error in"=w122, "idle state"=w129, "initial delay"=1e-09 ("Initial Delay")) -> ("task out"=w124:refnum<k21>, "error out"=w123:errorcluster)  [unwired: 3 in, 5 out]
          }
          frame Enabled {
          }
        }
        n28 = call-poly <vilib>:"DAQmx Timing.vi"("task/channels in"=w119, "sample mode"=w113, "samples per channel"=w112, "rate"=w111, "source"=w105, "error in"=w120) -> ("task out"=w108:refnum<k21>, "error out"=w109:errorcluster)  [unwired: 8 in]
        n29 = disable-structure shown="Enabled" {
          disable-tunnel: w109 -> [w137 w147]
          disable-tunnel: w108 -> [w136 w146]
          disable-tunnel: [w133 w146] -> w104
          disable-tunnel: [w132 w147] -> w103
          frame Disabled {
            n30 = call "Get Terminal Name with Device Prefix.vi"("error in (no error)"=w137, "Local Terminal Name"="Ctr0InternalOutput" ("terminal"), "task/channels in"=w136) -> ("error out"=w135:errorcluster, "Terminal Name with Device Prefix"=w131:tag, "task out"=w134:refnum<k21>)  [unwired: 1 in, 5 out]
            n31 = disable-structure shown="Enabled" {
              disable-tunnel: w135 -> [w143 w145]
              disable-tunnel: w134 -> [w142 w144]
              disable-tunnel: [w141 w144] -> w133
              disable-tunnel: [w140 w145] -> w132
              disable-tunnel: w131 -> [w139 _]
              frame Enabled {
                n32 = call-poly <vilib>:"DAQmx Trigger.vi"("task/channels in"=w142, "source"=w139, "error in"=w143) -> ("task out"=w141:refnum<k21>, "error out"=w140:errorcluster)  [unwired: 2 in, 9 out]
              }
              frame Disabled {
              }
            }
          }
          frame Enabled {
          }
        }
        n33 = property class="DAQmx Write"(reference=w104, error in=w103, "RegenMode"=w102) -> (reference out=w117:refnum<k21>, error out=w118:errorcluster)
      }
      frame "Write Scan Pattern" {
        n34 = call-poly <vilib>:"DAQmx Write.vi"("task/channels in"=w159, "auto start"=FALSE, "data"=w152, "error in"=w158) -> ("task out"=w153:refnum<k21>, "error out"=w151:errorcluster)  [unwired: 9 in, 1 out]
        n35 = call-poly <vilib>:"DAQmx Write.vi"("task/channels in"=w154, "auto start"=FALSE, "data"=w150, "error in"=w158) -> ("task out"=w155:refnum<k21>, "error out"=w157:errorcluster)  [unwired: 9 in, 1 out]
      }
      frame "Write DO only" {
        n36 = call-poly <vilib>:"DAQmx Write.vi"("task/channels in"=w164, "auto start"=FALSE, "data"=w163, "error in"=w160) -> ("task out"=w165:refnum<k21>, "error out"=w167:errorcluster)  [unwired: 9 in, 1 out]
      }
      frame "Start Galvo Task" {
        n37 = call <vilib>:"DAQmx Start Task.vi"("task/channels in"=w177, "error in"=w173) -> ("task out"=w176:refnum<k21>, "error out"=w172:errorcluster)  [unwired: 12 in]
        n38 = call <vilib>:"DAQmx Start Task.vi"("task/channels in"=w175, "error in"=w172) -> ("task out"=w174:refnum<k21>, "error out"=w170:errorcluster)  [unwired: 12 in]
        n39 = call <vilib>:"DAQmx Start Task.vi"("task/channels in"=w171, "error in"=w170) -> ("task out"=w168:refnum<k21>, "error out"=w169:errorcluster)  [unwired: 12 in]
      }
      frame "Start DO only" {
        n40 = call <vilib>:"DAQmx Start Task.vi"("task/channels in"=w188, "error in"=w184) -> ("task out"=w182:refnum<k21>, "error out"=w186:errorcluster)  [unwired: 12 in]
        n41 = disable-structure shown="Enabled" {
          disable-tunnel: w187 -> [w192 w194]
          disable-tunnel: w186 -> [w191 w193]
          disable-tunnel: [w190 w193] -> w180
          disable-tunnel: [w189 w194] -> w185
          frame Disabled {
            n42 = call <vilib>:"DAQmx Start Task.vi"("task/channels in"=w192, "error in"=w191) -> ("task out"=w189:refnum<k21>, "error out"=w190:errorcluster)  [unwired: 12 in]
          }
          frame Enabled {
          }
        }
        n43 = call <vilib>:"DAQmx Wait Until Done.vi"("task/channels in"=w182, "timeout (sec)"=20.0, "error in"=w180) -> ("task out"=w181:refnum<k21>, "error out"=w179:errorcluster)  [unwired: 11 in]
      }
      frame "Stop Galvo" {
        n44 = call <vilib>:"DAQmx Stop Task.vi"("task/channels in"=w202, "error in"=w198) -> ("task out"=w201:refnum<k21>, "error out"=w200:errorcluster)  [unwired: 12 in]
        n45 = call <vilib>:"DAQmx Stop Task.vi"("task/channels in"=w197, "error in"=w198) -> ("task out"=w196:refnum<k21>, "error out"=w195:errorcluster)  [unwired: 12 in]
        n46 = call <vilib>:"DAQmx Stop Task.vi"("task/channels in"=w204, "error in"=w198) -> ("task out"=w203:refnum<k21>, "error out"=w199:errorcluster)  [unwired: 12 in]
      }
      frame "Uninit" {
        n47 = call <vilib>:"DAQmx Clear Task.vi"("task in"=w211, "error in"=w209) -> ("error out"=w208:errorcluster)  [unwired: 13 in]
        n48 = call <vilib>:"DAQmx Clear Task.vi"("task in"=w210, "error in"=w208) -> ("error out"=w207:errorcluster)  [unwired: 13 in]
        n49 = call <vilib>:"DAQmx Clear Task.vi"("task in"=w205, "error in"=w207) -> ("error out"=w206:errorcluster)  [unwired: 13 in]
      }
      frame "Uninit DO only" {
        n50 = call <vilib>:"DAQmx Clear Task.vi"("task in"=w216, "error in"=w212) -> ("error out"=w215:errorcluster)  [unwired: 13 in]
        n51 = disable-structure shown="Enabled" {
          disable-tunnel: w215 -> [w219 w220]
          disable-tunnel: [w218 w220] -> w214
          disable-tunnel: w213 -> [w217 _]
          frame Disabled {
            n52 = call <vilib>:"DAQmx Clear Task.vi"("task in"=w217, "error in"=w219) -> ("error out"=w218:errorcluster)  [unwired: 13 in]
          }
          frame Enabled {
          }
        }
      }
      frame "Is Task Done?" {
        n53 = call <vilib>:"DAQmx Is Task Done.vi"("task/channels in"=w227, "error in"=w221) -> ("task out"=w223:refnum<k21>, "task done?"=w224:bool, "error out"=w226:errorcluster)  [unwired: 11 in]
        n54 = call <vilib>:"DAQmx Is Task Done.vi"("task/channels in"=w230, "error in"=w221) -> ("task out"=w229:refnum<k21>, "task done?"=w228:bool, "error out"=w222:errorcluster)  [unwired: 11 in]
        n55 = And(x=w224, y=w228) -> (x .and. y?=→"task done?":bool)
      }
    }
    n56 = Merge Errors(w18, w12, w6) -> (w19:errorcluster)
  }
  "error out" <- w4
